vi "Read Nest Actor Alias.vi"(7 "LVCAM":refnum<class "LVCAM.lvclass">) -> (0 "error out":errorcluster, 2 "Nest Actor Alias":string[](array[string]))   [LabVIEW 2021, in "LVCAM.lvlib" / "Self Actor.lvclass"]
uses:
  Self Actor.lvclass
  LVCAM/LVCAM.lvclass
  Self Actor.lvclass/Self Actor.ctl
  Msg Q/Msg Q.lvclass
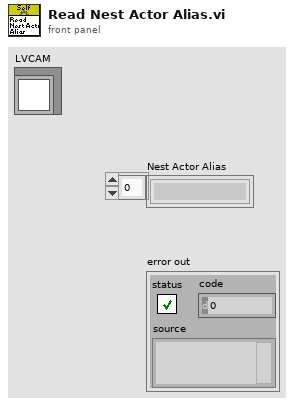
[diagram p1: front panel]
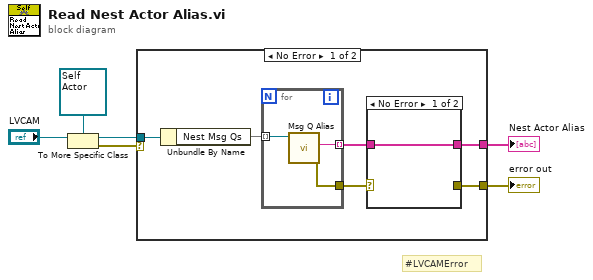
[diagram p0: block diagram]
diagram:
  # "#LVCAMError"
  n1 = To More Specific Class(target class=refnum<class "Self Actor.lvclass"> refnum ("LVCAM.lvlib:Self Actor.lvclass"), reference="LVCAM") -> (specific class reference=w3:refnum<class "Self Actor.lvclass">, error out=w1:errorcluster)  [unwired: 1 in]
  n2 = case shown="No Error" w1 {
    selector: w1 -> [_ w18]
    tunnel: [w9 w18] -> w6
    tunnel: [w8 _] -> w5
    tunnel: w3 -> [w11 _]
    frame No Error {
      n3 = Unbundle By Name(w11) -> ("Nest Msg Qs"=w12:set{refnum<class "Msg Q.lvclass">})
      n4 = for {
        tunnel: w12 -> [w17] mode=indexing
        tunnel: [w16] -> w7 mode=indexing
        tunnel: [w15] -> w10
        n5 = call "Msg Q Alias.vi"("Msg Q in"=w17) -> ("error out"=w15:errorcluster, "Msg Q Alias"=w16:string)  [unwired: 9 in]
      }
      n6 = case shown="No Error" w10 {
        selector: w10 -> [_ w14]
        tunnel: [_ w14] -> w9
        tunnel: [w13 _] -> w8
        tunnel: w7 -> [w13 _]
        frame No Error {
        }
        frame Error {
        }
      }
    }
    frame Error {
    }
  }
  "error out" <- w6
  "Nest Actor Alias" <- w5
